vi "str_initial_action_for_log_record.vi"(10 "path_Destin":path caption="Destination Folder", 11 "path_Orig":path caption="Original Files Folder") -> (3 "st_init_action_log_rec":string)   [LabVIEW 2026]
doc: "This subVI creates information from two path to log recods and documentation"
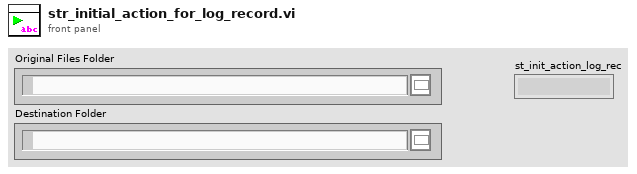
[diagram p1: front panel]
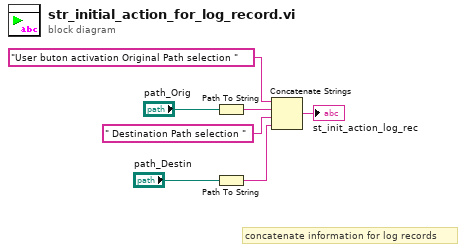
[diagram p0: block diagram]
diagram:
  # "concatenate information for log records"
  n1 = Path To String(path="path_Orig") -> (string=w4:string)
  n2 = Path To String(path="path_Destin") -> (string=w2:string)
  n3 = Concatenate Strings("User buton activation Original Path selection ", w4, " Destination Path selection ", w2) -> (→"st_init_action_log_rec":string)
